vi "Write Section.vi"(8 "error in (no error)":errorcluster, 10 "Section":string="Parameters", 11 "Analyze Parameter Base in":refnum<class "Analyze Parameter Base.lvclass">) -> (0 "error out":errorcluster, 3 "Analyze Parameter Base out":refnum<class "Analyze Parameter Base.lvclass">)   [LabVIEW 2020, in "Analyze Parameter Base.lvclass"]
uses:
  Analyze Parameter Base.lvclass
  Analyze Parameter Base.lvclass/Analyze Parameter Base.ctl
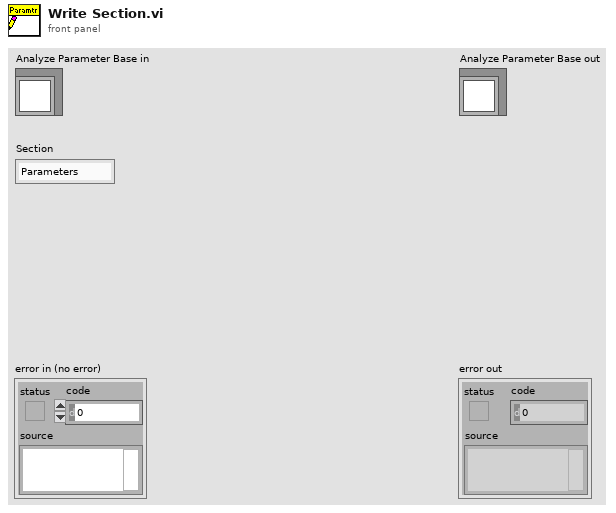
[diagram p1: front panel]
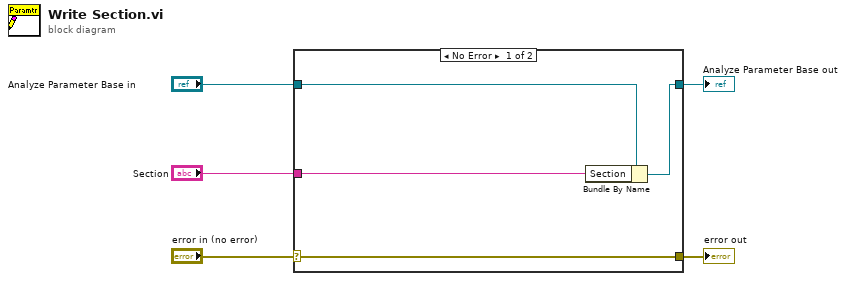
[diagram p0: block diagram]
diagram:
  n1 = case shown="No Error" "error in (no error)" {
    selector: "error in (no error)" -> [w9 w10]
    tunnel: [w9 w10] -> w4
    tunnel: [w7 w11] -> w2
    tunnel: "Analyze Parameter Base in" -> [w8 w11]
    tunnel: "Section" -> [w6 _]
    frame No Error {
      n2 = Bundle By Name(cluster=w8, "Section"=w6) -> (w7:refnum<class "Analyze Parameter Base.lvclass">)
    }
    frame Error {
    }
  }
  "error out" <- w4
  "Analyze Parameter Base out" <- w2
